vi "Periodic Tasks.vi"(8 "error in":errorcluster) -> ()   [LabVIEW 2023]
doc: "This VI runs in parallel to other tasks. It can contain as many user-defined periodic loops as you need. These can carry out PID or other sorts of timed response."
uses:
  <vilib>/Rock Robotics/WPI/Utilities/WPI_GetSetVariantRefNum.vi
  Robot Global Data.vi
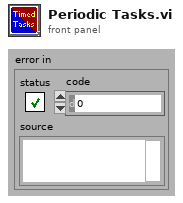
[diagram p1: front panel]
types:
  T1 = typedef "WPI_JoystickDevRef.ctl" = cluster{"Device":T2}
  T2 = typedef "WPI_JoystickDeviceEnum.ctl" = enum16{"USB 0", "USB 1", "USB 2", "USB 3", "USB 4", "USB 5"}
  T3 = typedef "WPI_RobotDriveDevRef.ctl" = cluster{"DevStatus":errorcluster, "Motors[]":T4[], "Square Inputs":bool, "Max Output":dbl}
  T4 = typedef "WPI_MotorControlDeviceRef.ctl" = cluster{"DeviceStatus":errorcluster, "Type":T5, "PWM":cluster{"PWM Channel":T6, "DeadBand":T7}, "CAN":cluster{"Device Number":u8, "SetOutput VI Ref":variant, "GetOutput VI Ref":variant, "Enable VI Ref":variant, "Disable VI Ref":variant, "Data":variant}, "Invert":bool, "DIO PWM":cluster{"PWM \"Enable\" Channel":T6, "DIOChannel":T8, "PWM Rate":dbl}}
  T5 = typedef "WPI_MotorControlType.ctl" = enum16{"PWM", "CAN", "DIO PWM"}
  T6 = typedef "FPGA_DIOPWMChannel.ctl" = enum8{"PWM 0", "PWM 1", "PWM 2", "PWM 3", "PWM 4", "PWM 5", "PWM 6", "PWM 7", "PWM 8", "PWM 9", "PWM MXP 0", "PWM MXP 1", "PWM MXP 2", "PWM MXP 3", "PWM MXP 4", "PWM MXP 5", "PWM MXP 6", "PWM MXP 7", "PWM MXP 8", "PWM MXP 9", "Invalid"}
  T7 = typedef "WPI_PWMDeadband.ctl" = cluster{"Name":string, "maxPositivePwm":i32, "minPositivePwm":i32, "centerPwm":i32, "maxNegativePwm":i32, "minNegativePwm":i32, "angularRange":u16}
  T8 = typedef "FPGA_DIOChannel.ctl" = enum8{"DIO 0", "DIO 1", "DIO 2", "DIO 3", "DIO 4", "DIO 5", "DIO 6", "DIO 7", "DIO 8", "DIO 9", "DIO MXP 0", "DIO MXP 1", "DIO MXP 2", "DIO MXP 3", "DIO MXP 4", "DIO MXP 5", "DIO MXP 6", "DIO MXP 7", "DIO MXP 8", "DIO MXP 9", "DIO MXP 10", "DIO MXP 11", "DIO MXP 12", "DIO MXP 13", "DIO MXP 14", "DIO MXP 15", "SPI Port CS1", "SPI Port CS2", "SPI Port CS3", "SPI Port MISO", "SPI Port MOSI", "Invalid"}
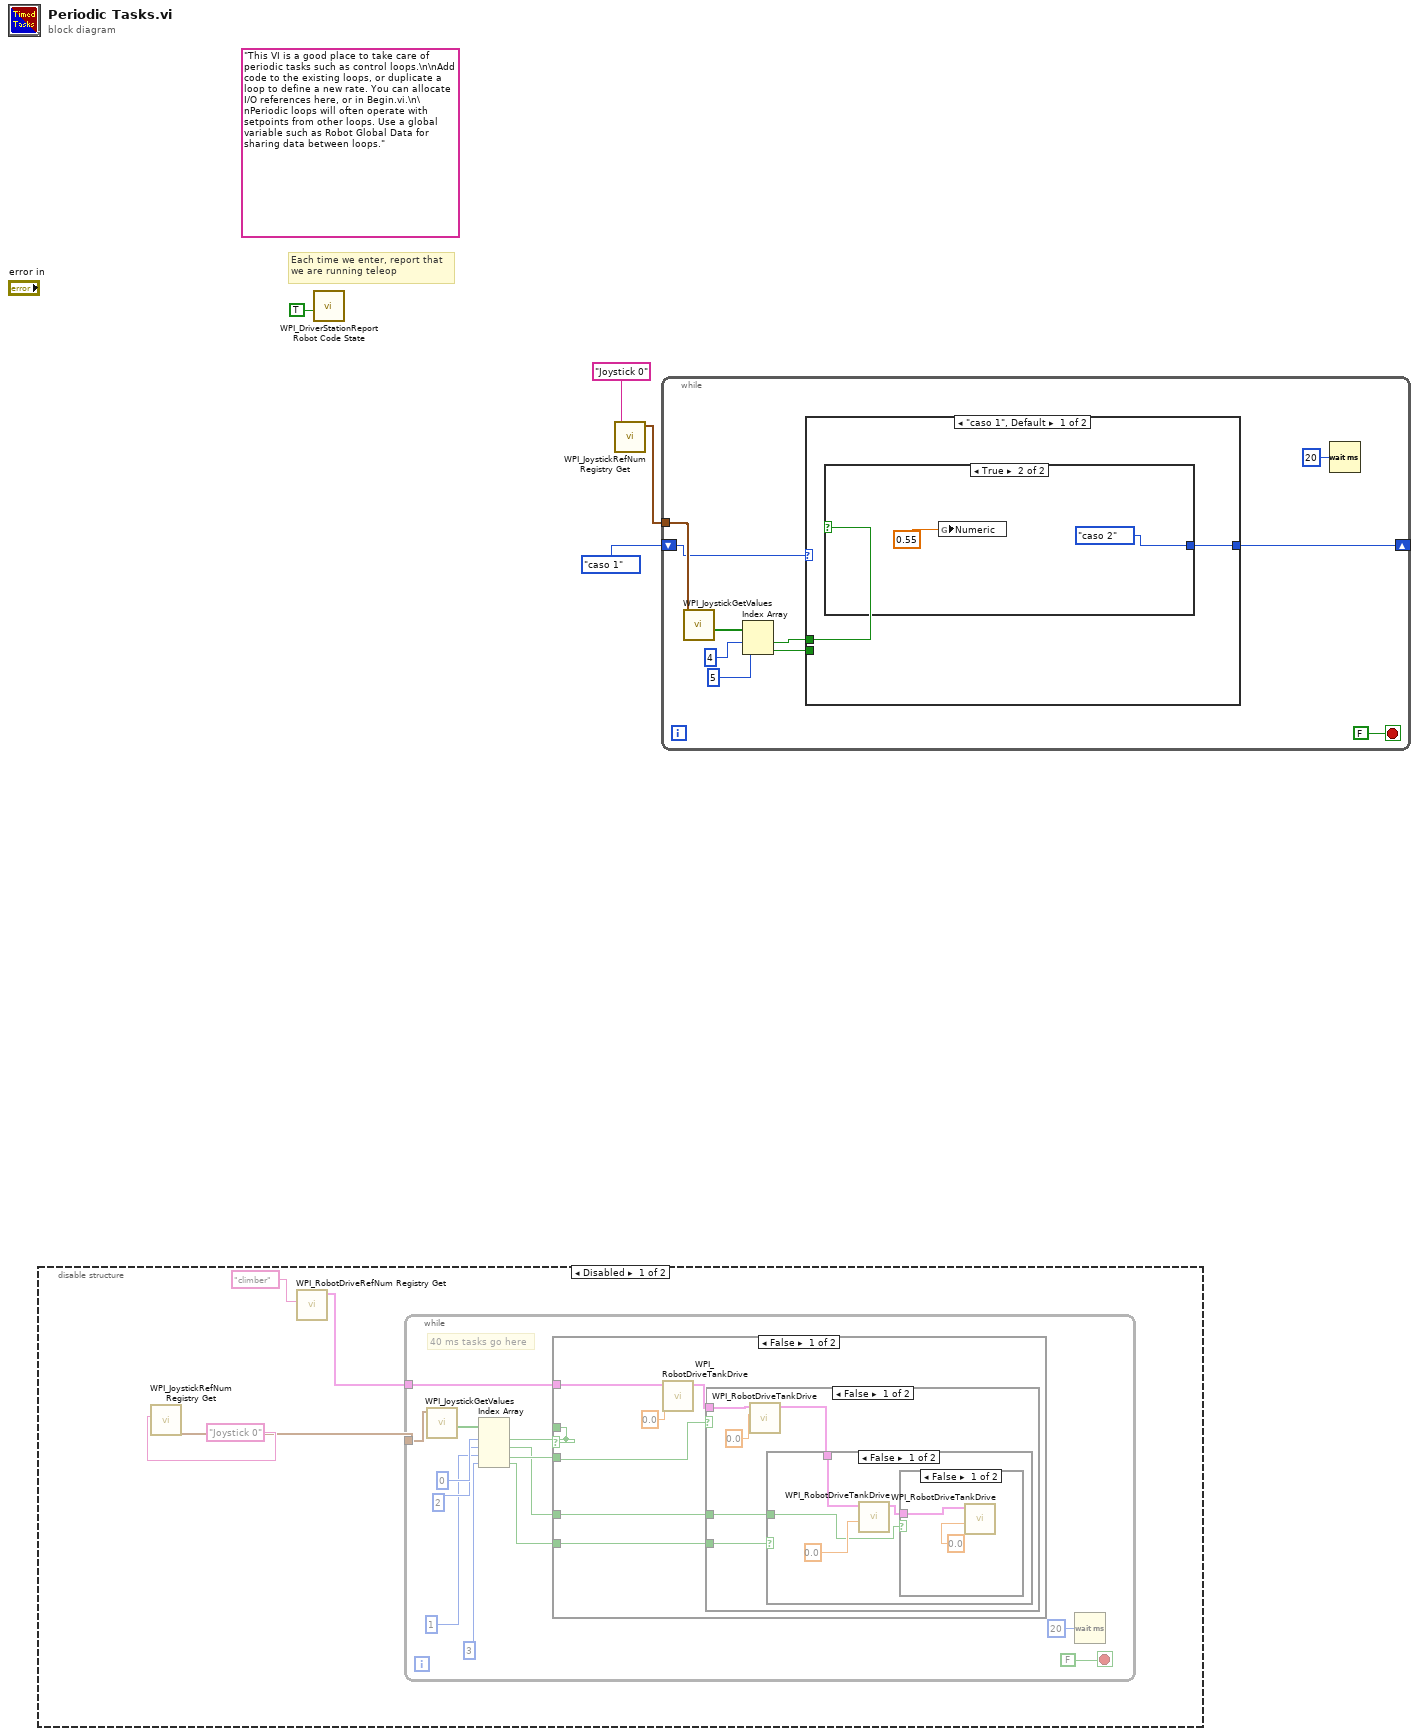
[diagram p0: block diagram]
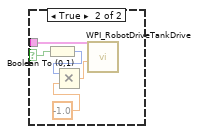
[diagram p2: hidden frame]
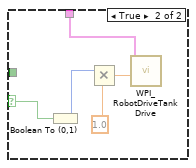
[diagram p3: hidden frame]
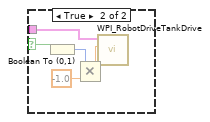
[diagram p4: hidden frame]
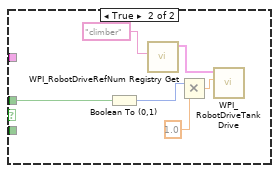
[diagram p5: hidden frame]
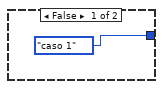
[diagram p7: hidden frame]
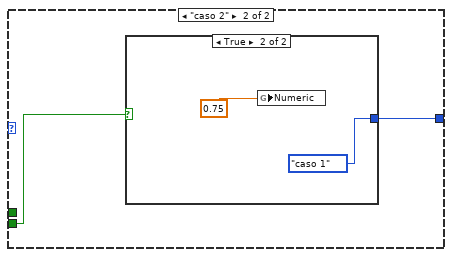
[diagram p8: hidden frame]
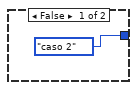
[diagram p9: hidden frame]
diagram:
  (unwired) "This VI is a good place to take care of periodic tasks such as control loops.\n\nAdd code to the existing loops, or duplicate a loop to define a new rate. You can allocate I/O references here, or in Begin.vi.\n\nPeriodic loops will often operate with setpoints from other loops. Use a global variable such as Robot Global Data for sharing data between loops."
  # "Each time we enter, report that\nwe are running teleop"
  n1 = disable-structure shown="Disabled" {
    frame Disabled {
      n2 = call <vilib>:"WPI_JoystickRefNum Registry Get.vi"("refnum name"="Joystick 0") -> ("JoystickDevRef"=w7:T1)  [unwired: 1 in, 9 out]
      n3 = call <vilib>:"WPI_RobotDriveRefNum Registry Get.vi"("refnum name"="climber") -> ("RobotDriveDevRef"=w5:T3)  [unwired: 1 in, 9 out]
      n4 = while {
        tunnel: w7 -> [w20]
        tunnel: w5 -> [w11]
        stop <- FALSE stop-if-true
        # "40 ms tasks go here"
        n5 = call <vilib>:"WPI_JoystickGetValues.vi"("JoystickDevRef"=w20) -> ("Buttons"=w18:bool[])  [unwired: 6 in, 4 out]
        n6 = Index Array(array=w18, index #1=0 ("index"), index #2=2 ("index"), index #3=1 ("index"), index #4=3 ("index")) -> (element #1=w12:bool, element #2=w9:bool, element #3=w15:bool, element #4=w10:bool)
        n7 = case shown="False" w12 {
          tunnel: w15 -> [w26 _]
          tunnel: w12 -> [_ w56]
          tunnel: w11 -> [w24 _]
          tunnel: w10 -> [w23 _]
          tunnel: w9 -> [w22 _]
          frame False {
            n8 = call <vilib>:"WPI_RobotDriveTankDrive.vi"("Left axis value"=0.0, "RobotDriveDevRef"=w24) -> ("RobotDriveDevRef"=w25:T3)  [unwired: 7 in, 2 out]
            n9 = case shown="False" w26 {
              selector: w26 -> [_ w52]
              tunnel: w25 -> [w32 w53]
              tunnel: w23 -> [w29 _]
              tunnel: w22 -> [w28 _]
              frame False {
                n10 = call <vilib>:"WPI_RobotDriveTankDrive.vi"("Left axis value"=0.0, "RobotDriveDevRef"=w32) -> ("RobotDriveDevRef"=w30:T3)  [unwired: 7 in, 2 out]
                n11 = case shown="False" w29 {
                  selector: w29 -> [_ w48]
                  tunnel: w30 -> [w34 w44]
                  tunnel: w28 -> [w33 _]
                  frame False {
                    n12 = call <vilib>:"WPI_RobotDriveTankDrive.vi"("Right axis value"=0.0 ("Left axis value"), "RobotDriveDevRef"=w34) -> ("RobotDriveDevRef"=w35:T3)  [unwired: 7 in, 2 out]
                    n13 = case shown="False" w33 {
                      selector: w33 -> [_ w41]
                      tunnel: w35 -> [w38 w43]
                      frame False {
                        n14 = call <vilib>:"WPI_RobotDriveTankDrive.vi"("Right axis value"=0.0 ("Left axis value"), "RobotDriveDevRef"=w38) -> ()  [unwired: 7 in, 3 out]
                      }
                      frame True {
                        n15 = Boolean To (0,1)(Boolean=w41) -> (0, 1=w40:i16)
                        n16 = Multiply(x=w40, y=-1.0) -> (x*y=w39:dbl)
                        n17 = call <vilib>:"WPI_RobotDriveTankDrive.vi"("Right axis value"=w39, "RobotDriveDevRef"=w43) -> ()  [unwired: 7 in, 3 out]
                      }
                    }
                  }
                  frame True {
                    n18 = Boolean To (0,1)(Boolean=w48) -> (0, 1=w47:i16)
                    n19 = Multiply(x=w47, y=1.0 ("Left axis value")) -> (x*y=w45:dbl)
                    n20 = call <vilib>:"WPI_RobotDriveTankDrive.vi"("Right axis value"=w45, "RobotDriveDevRef"=w44) -> ()  [unwired: 7 in, 3 out]
                  }
                }
              }
              frame True {
                n21 = Boolean To (0,1)(Boolean=w52) -> (0, 1=w51:i16)
                n22 = Multiply(x=w51, y=-1.0) -> (x*y=w49:dbl)
                n23 = call <vilib>:"WPI_RobotDriveTankDrive.vi"("Left axis value"=w49, "RobotDriveDevRef"=w53) -> ()  [unwired: 7 in, 3 out]
              }
            }
          }
          frame True {
            n24 = Boolean To (0,1)(Boolean=w56) -> (0, 1=w59:i16)
            n25 = call <vilib>:"WPI_RobotDriveRefNum Registry Get.vi"("refnum name"="climber") -> ("RobotDriveDevRef"=w55:T3)  [unwired: 1 in, 9 out]
            n26 = Multiply(x=w59, y=1.0 ("Left axis value")) -> (x*y=w57:dbl)
            n27 = call <vilib>:"WPI_RobotDriveTankDrive.vi"("Left axis value"=w57, "RobotDriveDevRef"=w55) -> ()  [unwired: 7 in, 3 out]
          }
        }
        n28 = Wait (ms)(milliseconds to wait=u32 20) -> ()  [unwired: 1 out]
      }
    }
    frame Enabled {
    }
  }
  n29 = call <vilib>:"WPI_DriverStationReport Robot Code State.vi"("TeleOp"=TRUE ("Autonomous")) -> ()  [unwired: 10 in, 1 out]
  n30 = call <vilib>:"WPI_JoystickRefNum Registry Get.vi"("refnum name"="Joystick 0") -> ("JoystickDevRef"=w3:T1)  [unwired: 9 in, 1 out]
  n31 = while {
    tunnel: w3 -> [w68]
    shift-right: [w61] -> _
    shift-left: enum16{"caso 1", "caso 2"}."caso 1" -> [w64]
    stop <- FALSE stop-if-true
    n32 = call <vilib>:"WPI_JoystickGetValues.vi"("JoystickDevRef"=w68) -> ("Buttons"=w67:bool[])  [unwired: 6 in, 4 out]
    n33 = Index Array(array=w67, index #1=4 ("index"), index #2=5 ("index")) -> (element #1=w63:bool, element #2=w62:bool)
    n34 = case shown="\"caso 1\", Default" w64 {
      tunnel: w63 -> [w71 _]
      tunnel: w62 -> [_ w76]
      tunnel: [w70 w75] -> w61
      frame "caso 1", Default {
        n35 = case shown="True" w71 {
          tunnel: [enum16{"caso 1", "caso 2"}."caso 1" enum16{"caso 1", "caso 2"}."caso 2"] -> w70
          frame False {
          }
          frame True {
            n36 = global write "Robot Global Data.vi" "Numeric"(0.55) -> ()
          }
        }
      }
      frame "caso 2" {
        n37 = case shown="True" w76 {
          tunnel: [enum16{"caso 1", "caso 2"}."caso 2" enum16{"caso 1", "caso 2"}."caso 1"] -> w75
          frame False {
          }
          frame True {
            n38 = global write "Robot Global Data.vi" "Numeric"(0.75) -> ()
          }
        }
      }
    }
    n39 = Wait (ms)(milliseconds to wait=u32 20) -> ()  [unwired: 1 out]
  }
